vi "MotorController.vi"(6 "stop":bool, 8 "X Velocity (m/s)":dbl(slide) min=-1.0 max=1.0 scale=-1.0..1.0, 11 "Y Velocity (m/s)":dbl(slide) min=-1.0 max=1.0 scale=-1.0..1.0) -> ()   [LabVIEW 2012]
uses:
  <vilib>/robotics/Steering/Wheel/Wheel Parameters.ctl
  <vilib>/robotics/Steering/Wheel/Rotation Direction.ctl
  <vilib>/robotics/Steering/Mecanum Wheel/Create Mecanum Wheel.vi
  <vilib>/robotics/Steering/Mecanum Steering Frame/Create Mecanum Steering Frame.vi
  <vilib>/robotics/Steering/Steering Frame/Apply Steering Frame Velocity to Wheels.vi
  <vilib>/robotics/Steering/Wheel/NI_Robotics_Wheel.lvclass
  <vilib>/robotics/Steering/Mecanum Wheel/NI_Robotics_Mecanum Wheel.lvclass
  <vilib>/robotics/Steering/Steering Frame/NI_Robotics_Steering Frame.lvclass
  <vilib>/robotics/Steering/Mecanum Steering Frame/NI_Robotics_Mecanum Steering Frame.lvclass
panel:
  out "Front Left":dbl format="%#.2g"
  out "Front Right":dbl format="%#.2g"
  out "Rear Left":dbl format="%#.2g"
  out "Rear Right":dbl format="%#.2g"
  in  "Angular Velocity (rad/s)":dbl(slide) min=-1.0 max=1.0 scale=1.0..-1.0
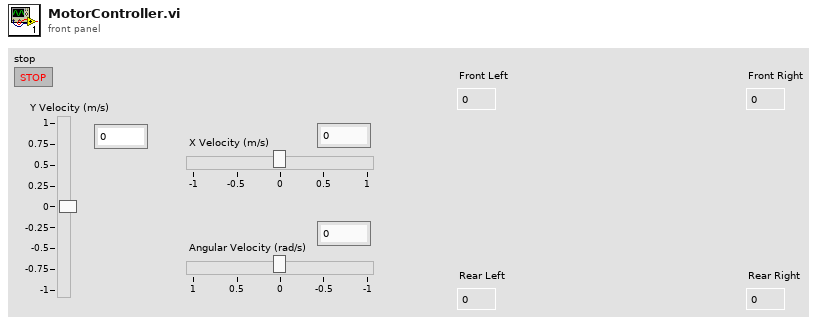
[diagram p1: front panel]
types:
  T1 = typedef "NI_Robotics_Wheel.lvclass/Wheel Parameters.ctl" = cluster{"wheel radius":dbl, "gear ratio":dbl, "forward rotation direction":T2}
  T2 = typedef "NI_Robotics_Wheel.lvclass/Rotation Direction.ctl" = u16
  T3 = cluster{"mecanum wheel out":refnum<class "NI_Robotics_Mecanum Wheel.lvclass">, "mecanum wheel out":refnum<class "NI_Robotics_Mecanum Wheel.lvclass">, "mecanum wheel out":refnum<class "NI_Robotics_Mecanum Wheel.lvclass">, "mecanum wheel out":refnum<class "NI_Robotics_Mecanum Wheel.lvclass">}
  T4 = typedef "NI_Robotics_Wheel.lvclass/Wheel State.ctl" = cluster{"wheel name":string, "forward angular velocity":dbl, "caster angular velocity":dbl, "caster wheel angle (rad)":dbl, "steering angle (rad)":dbl}
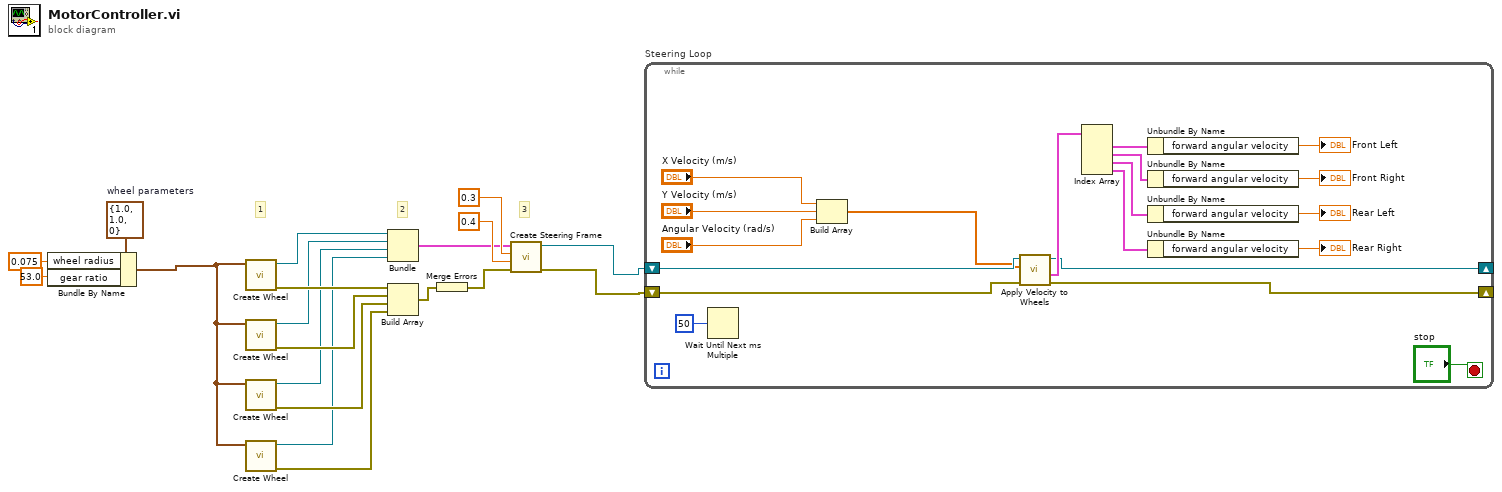
[diagram p0: block diagram]
diagram:
  w4 = T1 {"wheel radius"=1.0, "gear ratio"=1.0, "forward rotation direction"=0}  # wheel parameters
  # "3"
  # "2"
  # "1"
  n1 = Bundle By Name(cluster=w4, "wheel radius"=0.075, "gear ratio"=53.0) -> (w3:T1)
  n2 = call-poly <vilib>:"Create Wheel.vi"("wheel parameters"=w3) -> ("error out"=w14:errorcluster, "mecanum wheel out"=w7:refnum<class "NI_Robotics_Mecanum Wheel.lvclass">)  [unwired: 9 in]
  n3 = call-poly <vilib>:"Create Wheel.vi"("wheel parameters"=w3) -> ("error out"=w15:errorcluster, "mecanum wheel out"=w8:refnum<class "NI_Robotics_Mecanum Wheel.lvclass">)  [unwired: 9 in]
  n4 = call-poly <vilib>:"Create Wheel.vi"("wheel parameters"=w3) -> ("error out"=w16:errorcluster, "mecanum wheel out"=w9:refnum<class "NI_Robotics_Mecanum Wheel.lvclass">)  [unwired: 9 in]
  n5 = call-poly <vilib>:"Create Wheel.vi"("wheel parameters"=w3) -> ("error out"=w18:errorcluster, "mecanum wheel out"=w10:refnum<class "NI_Robotics_Mecanum Wheel.lvclass">)  [unwired: 9 in]
  n6 = Bundle("mecanum wheel out"=w7, "mecanum wheel out"=w8, "mecanum wheel out"=w9, "mecanum wheel out"=w10) -> (w11:T3)  [unwired: 1 in]
  n7 = Build Array(w14, w15, w16, w18) -> (w17:errorcluster[])
  n8 = Merge Errors(w17) -> (w19:errorcluster)
  n9 = call-poly <vilib>:"Create Steering Frame.vi"("error in (no error)"=w19, "wheel separation length"=0.4, "wheel separation width"=0.3, "wheels"=w11) -> ("error out"=w1:errorcluster, "mecanum steering frame out"=w2:refnum<class "NI_Robotics_Mecanum Steering Frame.lvclass">)  [unwired: 6 in]
  n10 = while "Steering Loop" {
    shift-right: [w22] -> _
    shift-left: w2 -> [w34]
    shift-right: [w21] -> _
    shift-left: w1 -> [w32]
    stop <- "stop" stop-if-true
    n11 = Wait Until Next ms Multiple(millisecond multiple=u32 50) -> ()  [unwired: 1 out]
    n12 = Build Array("X Velocity (m/s)", "Y Velocity (m/s)", "Angular Velocity (rad/s)") -> (w33:dbl[])
    n13 = call-poly <vilib>:"Apply Velocity to Wheels.vi"("error in (no error)"=w32, "steering frame velocity"=w33, "steering frame in"=w34) -> ("error out"=w21:errorcluster, "calculated wheel states"=w23:T4[], "steering frame out"=w22:refnum<class "NI_Robotics_Mecanum Steering Frame.lvclass">)  [unwired: 5 in, 1 out]
    n14 = Index Array(array=w23) -> (element #1=w24:T4, element #2=w27:T4, element #3=w26:T4, element #4=w25:T4)  [unwired: 4 in]
    n15 = Unbundle By Name(w24) -> ("forward angular velocity"=→"Front Left":dbl)
    n16 = Unbundle By Name(w27) -> ("forward angular velocity"=→"Front Right":dbl)
    n17 = Unbundle By Name(w26) -> ("forward angular velocity"=→"Rear Left":dbl)
    n18 = Unbundle By Name(w25) -> ("forward angular velocity"=→"Rear Right":dbl)
  }
